vi "main.vi"() -> ()   [LabVIEW 2021]
uses:
  Sources/Plotting-Axis.ctl
  VNA_DataType.ctl
  GEN_States.ctl
  Sources/Data_Cluster.ctl
  Sources/Measurement_Cluster.ctl
  Sources/Mode_Enum.ctl
  Library/TerminalDef.ctl
  <vilib>/Utility/config.llb/Config Data RefNum.ctl
  e59eb776-c2e1-4916-866f-0ee3ec66ac1c.vi
  <vilib>/Utility/config.llb/NI_LVConfig.lvlib
  Library/LibDan.lvlib
panel:
  in  "Control Tab":enum32{"General"}(tab)
  in  "S22Param":enum16{"S11", "S21", "S12", "S22"}(ring)=enum."S22"
  in  "S12Param":enum16{"S11", "S21", "S12", "S22"}(ring)=enum."S12"
  in  "S21Param":enum16{"S11", "S21", "S12", "S22"}(ring)=enum."S21"
  in  "Ramp Dir.":bool=TRUE
  in  "End B (T)":dbl
  in  "Delta B (T)":dbl
  in  "1/s":dbl
  in  "Measure Mode":enum32{"Deltat", "DeltaT", "dB"}(radio)
  in  "Stop @ T/B":bool=TRUE
  out "Temperature (K)":dbl
  out "Mag. Field (T)":dbl
  in  "Log Prefix":string="VNALog"
  in  "Data Type S22":T1
  in  "Data Type S12":T1
  in  "Data Type S21":T1
  in  "Data Type S11":T1
  in  "S22Bool":bool
  in  "S12Bool":bool
  in  "S21Bool":bool
  in  "S11Bool":bool
  in  "End T (K)":dbl
  in  "Delta T (K)":dbl
  in  "StopM_Button":bool
  in  "Log_Button":bool
  in  "Measure_Button":bool
  out "Global B":bool
  out "Global T":bool
  out "Logging":bool
  out "Measuring":bool
  in  "Global T VarRef":refnum<k21>
  in  "Global B VarRef":refnum<k21>
  in  "S11Param":enum16{"S11", "S21", "S12", "S22"}(ring)
  in  "Display Tab":T2(tab)
  out "Terminal":string
  in  "Clear_Button":bool
  in  "Y-Axis":T3=enum."Temperature"
  in  "X-Axis":T3
  out "Test Graph":cluster{"X":dbl, "Y":dbl}[](graph)
  in  "Max Elements":i32=5000
  out "Parameter Plots":cluster{"Ramp Pattern":dbl[], "VNA S22":dbl[]}(graph)
  in  "Param":enum16{"S11", "S21", "S12", "S22"}(ring)
  in  "Following":enum32{"Mag", "Temp", "Last"}(radio)=enum."Last"
  in  "Exit_Button":bool
  # "Parameter"
  # "Data Type"
  # "On/Off"
  # "S12"
  # "S22"
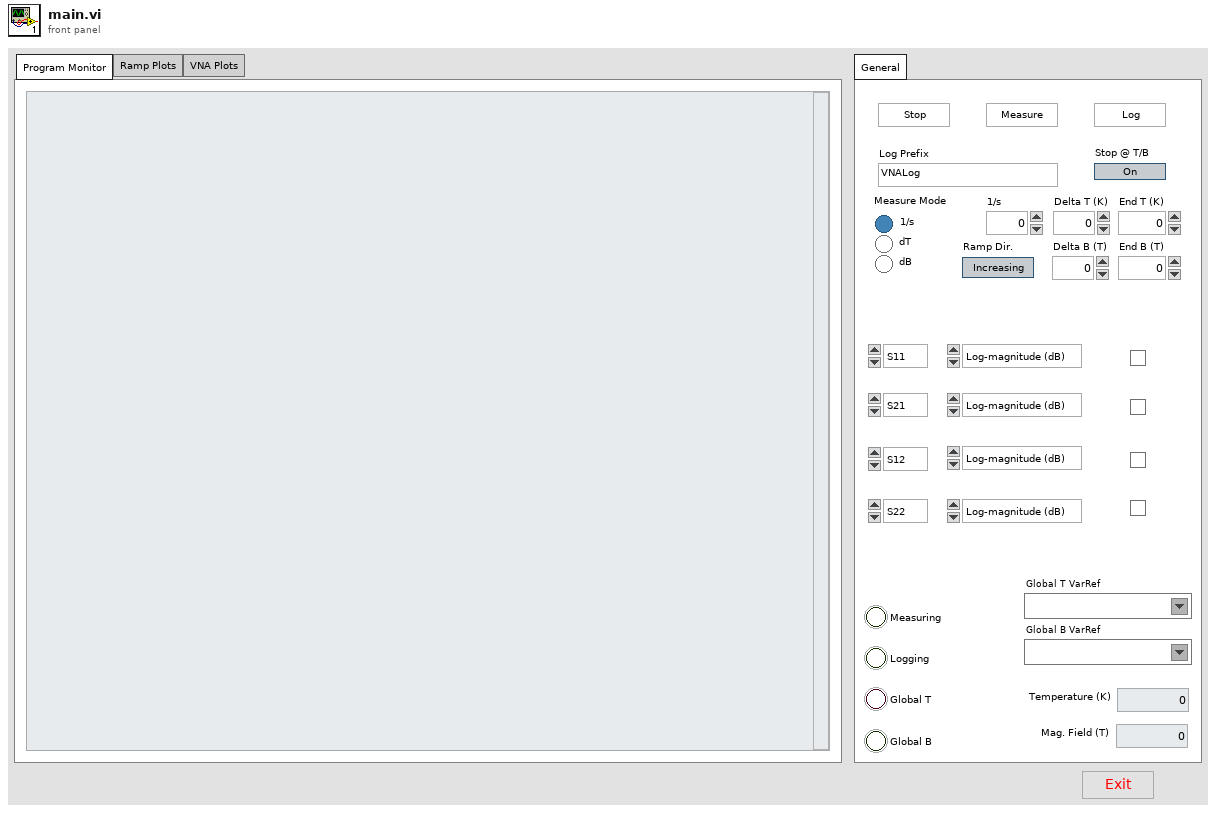
[diagram p1: front panel]
types:
  T1 = typedef "VNA_DataType.ctl" = enum16{"Log-magnitude (dB)", "Linear magnitude", "Phase (deg)", "Time Domain", "Real", "Imaginary", "Group Delay", "Polarlinear"}
  T2 = enum32{"Program Monitor", "Ramp Plots", "VNA Plots"}
  T3 = typedef "Plotting-Axis.ctl" = enum16{"Time", "Temperature", "Magnetic Field"}
  T4 = cluster{"Name":string, "Map":map{string, string}}
  T5 = typedef "LibDan.lvlib/TerminalDef.ctl" = cluster{"Terminal":cluster{"Data":string, "Prompt":string, "Output Refnum":refnum<vi>, "Input":string, "Input Refnum":refnum<vi>}, "TCP":cluster{"HostIP":string, "ServiceName":string, "Port":u16, "Timeout":i32, "TCP ID":refnum<k5>, "TCPConID":refnum<k5>, "Listening?":bool, "ClientCon?":bool}, "Config":cluster{"Path":path, "PathRef":T6, "NewFile?":bool, "Sections":cluster{"Name":string, "Map":map{string, string}}[]}}
  T6 = typedef "NI_LVConfig.lvlib/Config Data RefNum.ctl" = refnum<k1>
  T7 = typedef "Data_Cluster.ctl" = cluster{"Value":dbl, "GUI Data Cluster":cluster{"S11":bool, "S21":bool, "S12":bool, "S22":bool, "S11Meas":enum16{"Log-magnitude (dB)", "Linear magnitude", "Phase (deg)", "Time Domain", "Real", "Imaginary", "Group Delay", "Polarlinear"}, "S21Meas":enum16{"Log-magnitude (dB)", "Linear magnitude", "Phase (deg)", "Time Domain", "Real", "Imaginary", "Group Delay", "Polarlinear"}, "S12Meas":enum16{"Log-magnitude (dB)", "Linear magnitude", "Phase (deg)", "Time Domain", "Real", "Imaginary", "Group Delay", "Polarlinear"}, "S22Meas":enum16{"Log-magnitude (dB)", "Linear magnitude", "Phase (deg)", "Time Domain", "Real", "Imaginary", "Group Delay", "Polarlinear"}, "S11Param":enum16{"S11", "S21", "S12", "S22"}, "S21Param":enum16{"S11", "S21", "S12", "S22"}, "S12Param":enum16{"S11", "S21", "S12", "S22"}, "S22Param":enum16{"S11", "S21", "S12", "S22"}}, "Timing":cluster{"Last Operation":dbl, "Stop @ T/B":bool, "Last Temp":dbl, "Last Mag":dbl, "Ramp Param":cluster{"End T (K)":dbl, "Delta T (K)":dbl, "End B (T)":dbl, "Delta B (T)":dbl}, "LastOp?":bool, "FirstOp?":bool}, "Measurements":T8[], "Hardware":cluster{"VNA TCP Con":refnum<k5>, "VNA TCP Port":i32, "Global T VAR":refnum<k21>, "Global B VAR":refnum<k21>}, "Operation":cluster{"Operation Mode":T9, "Log Folder":path, "Measure Mode":enum32{"Deltat", "DeltaT", "dB"}}}
  T8 = typedef "Measurement_Cluster.ctl" = cluster{"Time Stamp":timestamp, "Temp T":dbl, "Mag B":dbl, "VNA S11":dbl[], "VNA S21":dbl[], "VNA S12":dbl[], "VNA S22":dbl[], "SweepParamArray":cluster{"Start f":dbl, "Stop f":dbl, "Pnts":i32, "Step f":dbl}[]}
  T9 = typedef "Mode_Enum.ctl" = enum16{"Logging", "Idle-Off", "Idle"}
  T10 = typedef "GEN_States.ctl" = enum16{"ClearBuffers", "SwitchToMeas", "SwitchToLog", "SwitchToOff", "Disconnect", "ExitSafe", "RefreshPlotMUnits", "UpdatePlots", "RefreshMUnits", "Read/WriteAll", "InitGUI", "Idle", "ProgInit", "Connect", "ConnectFail"}
  T11 = cluster{"Name":string, "Map":map{string, string}}[]
  T12 = enum16{"Standard", "Buffered", "CRLF", "Immediate"}
  T13 = cluster{"End T (K)":dbl, "Delta T (K)":dbl, "End B (T)":dbl, "Delta B (T)":dbl}
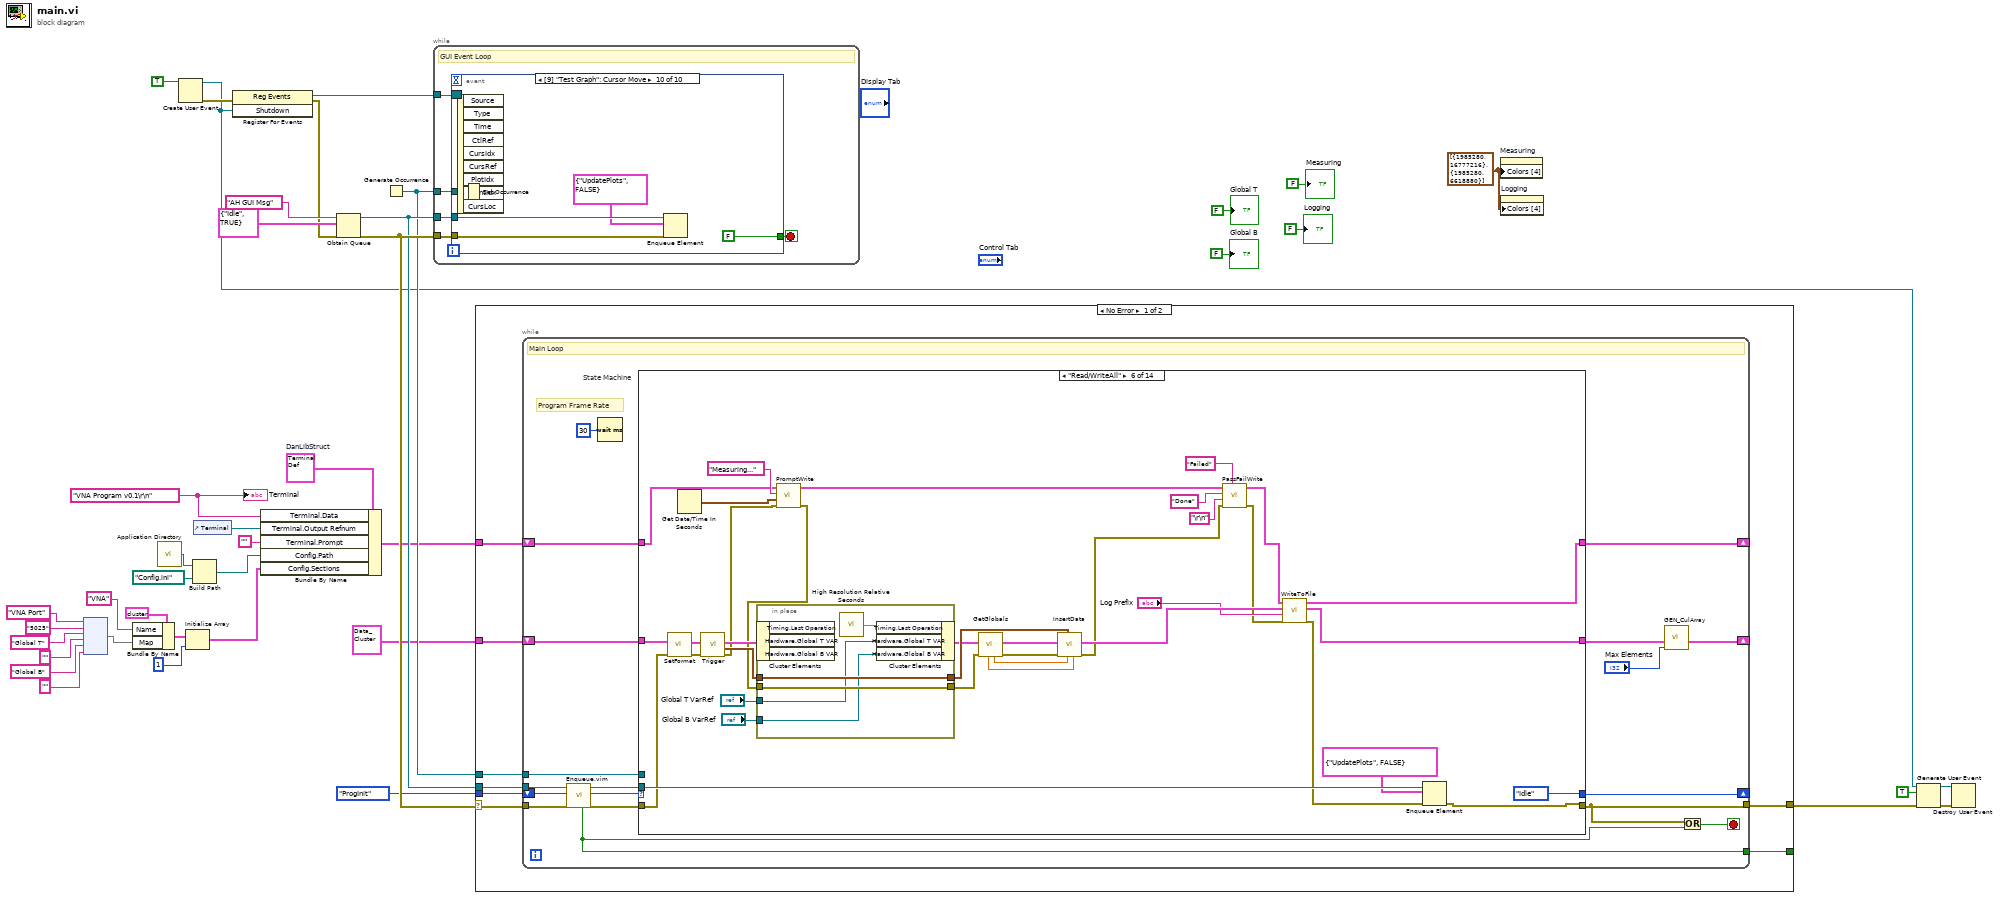
[diagram p0: block diagram]
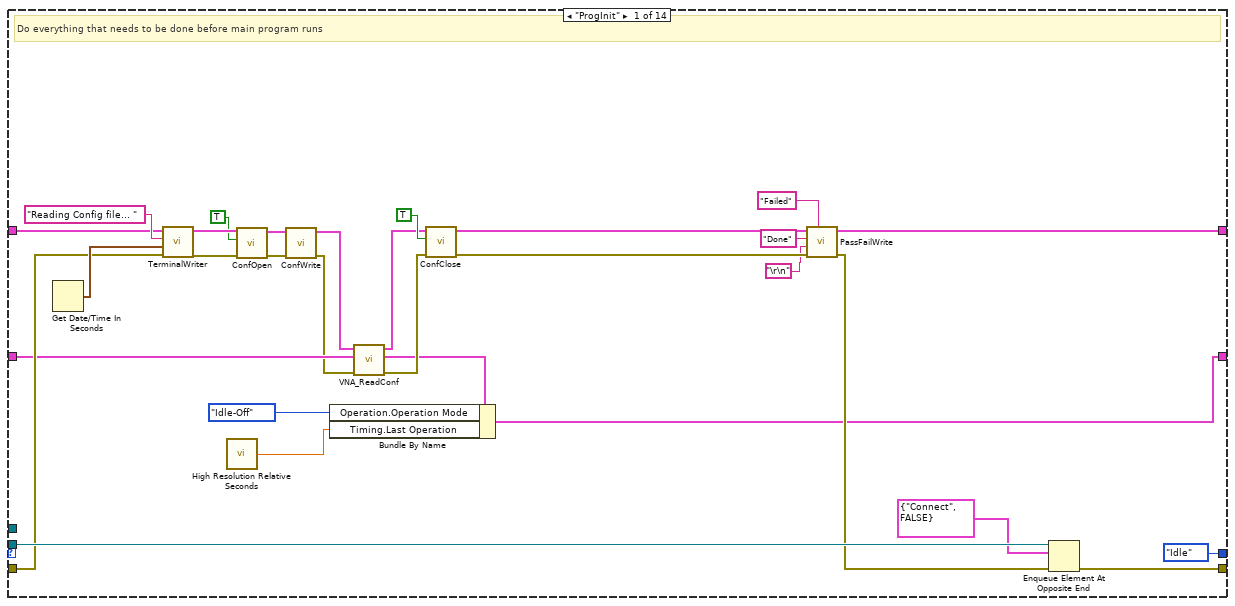
[diagram p2: hidden frame]
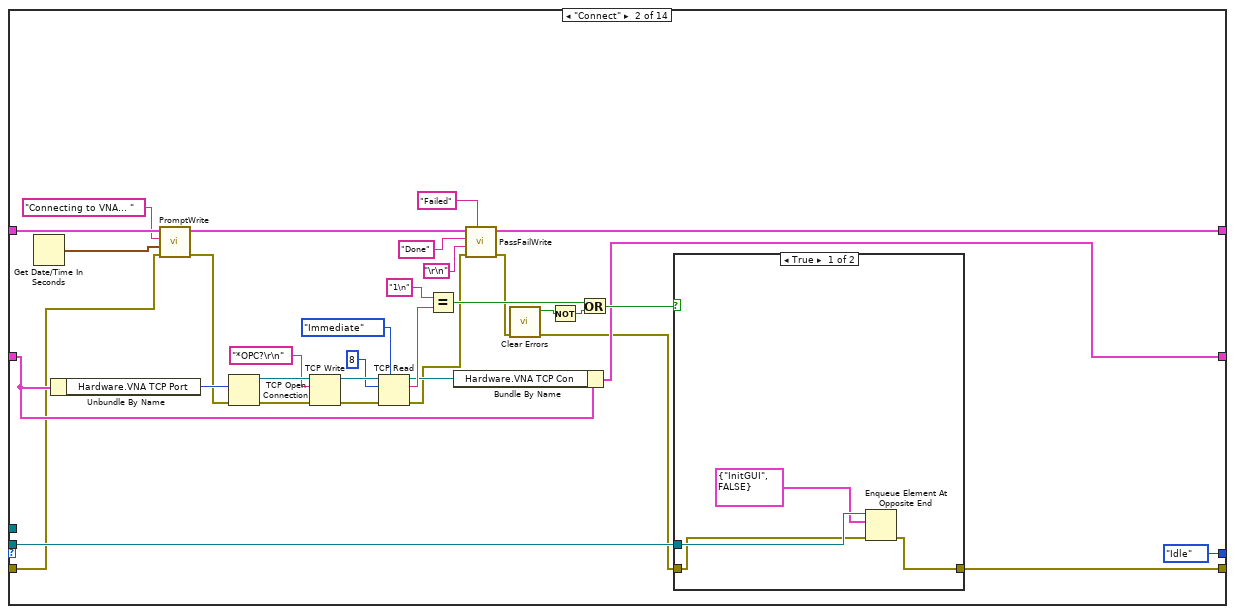
[diagram p3: hidden frame]
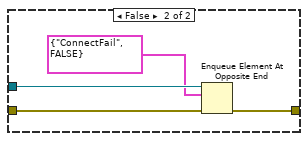
[diagram p4: hidden frame]
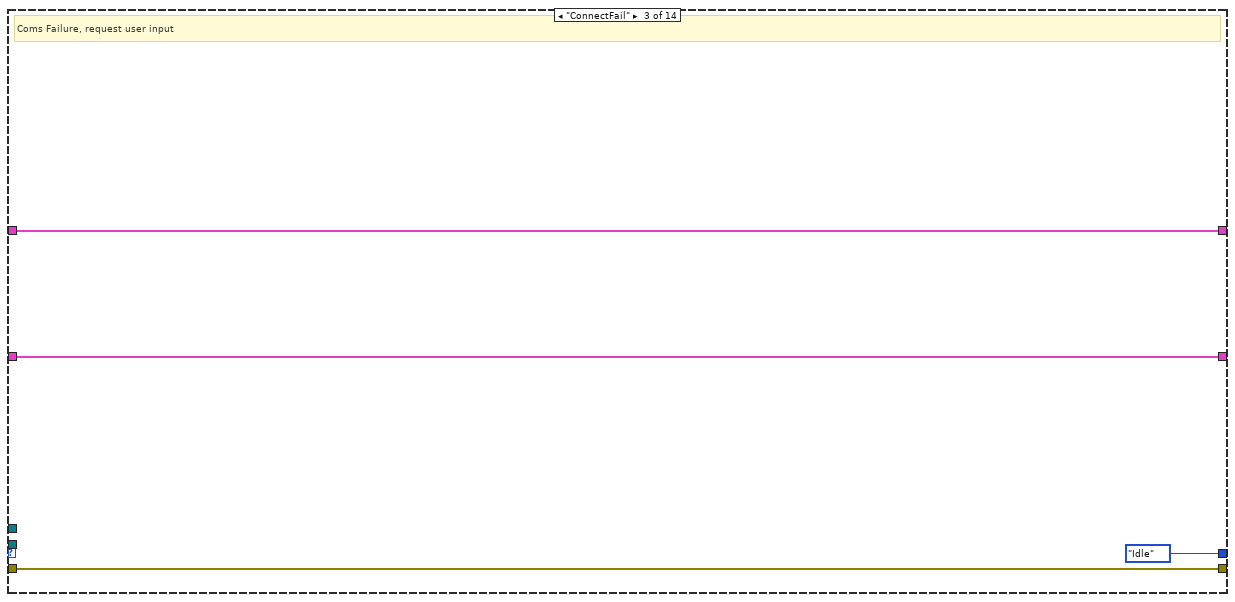
[diagram p5: hidden frame]
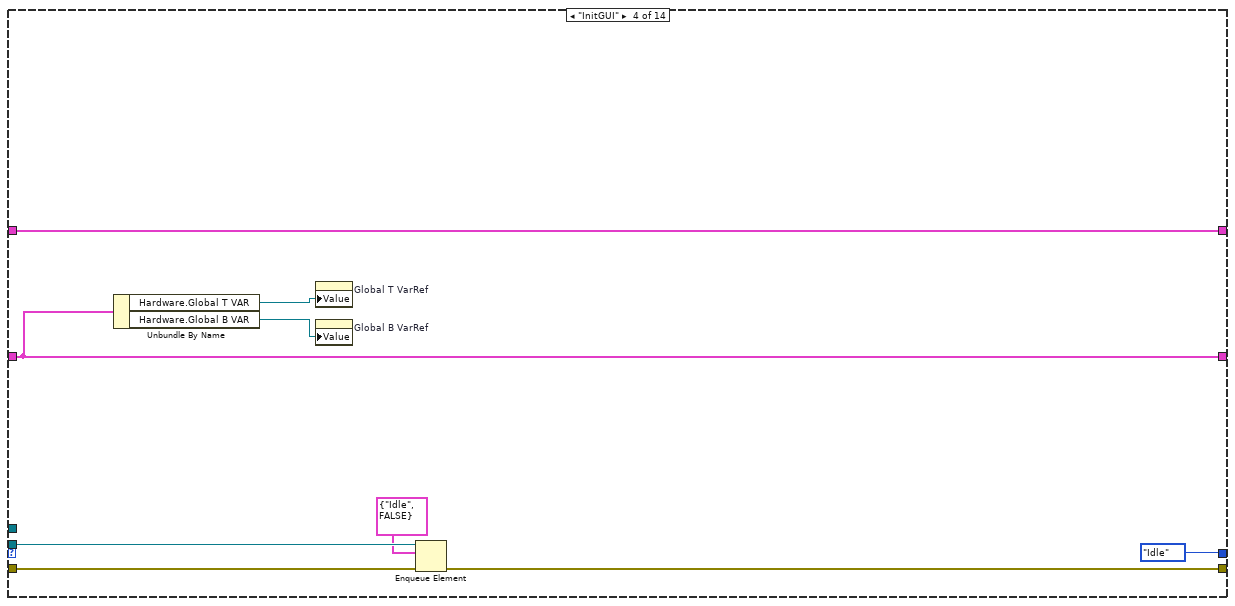
[diagram p6: hidden frame]
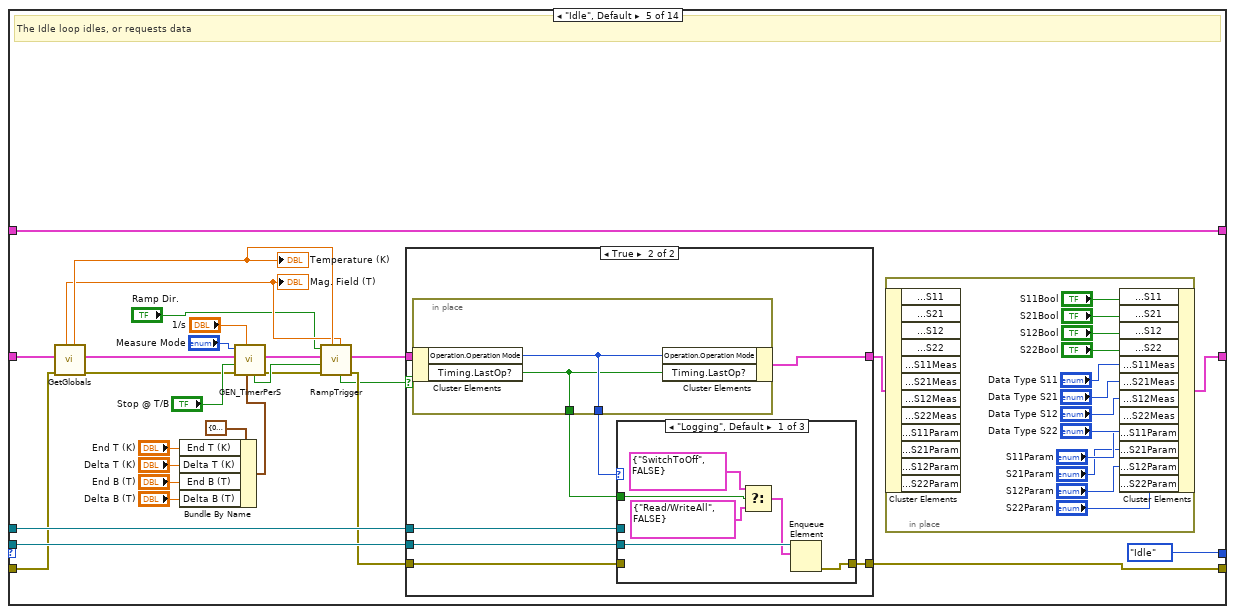
[diagram p7: hidden frame]
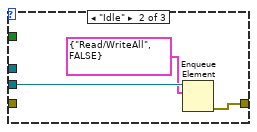
[diagram p9: hidden frame]
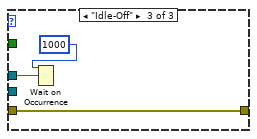
[diagram p10: hidden frame]
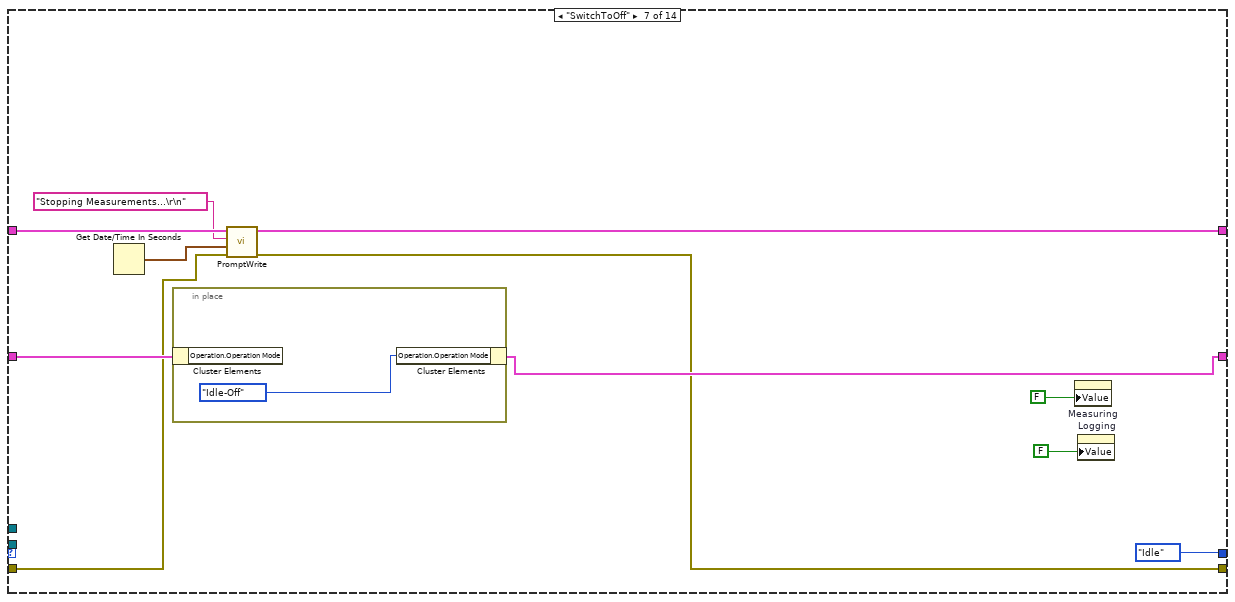
[diagram p11: hidden frame]
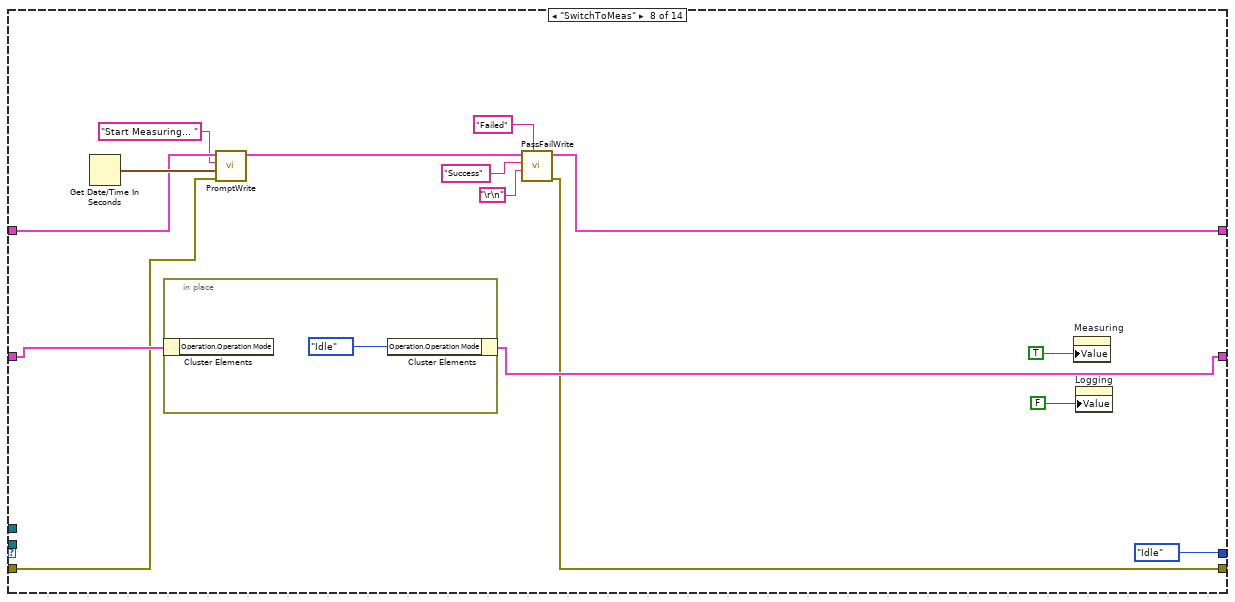
[diagram p12: hidden frame]
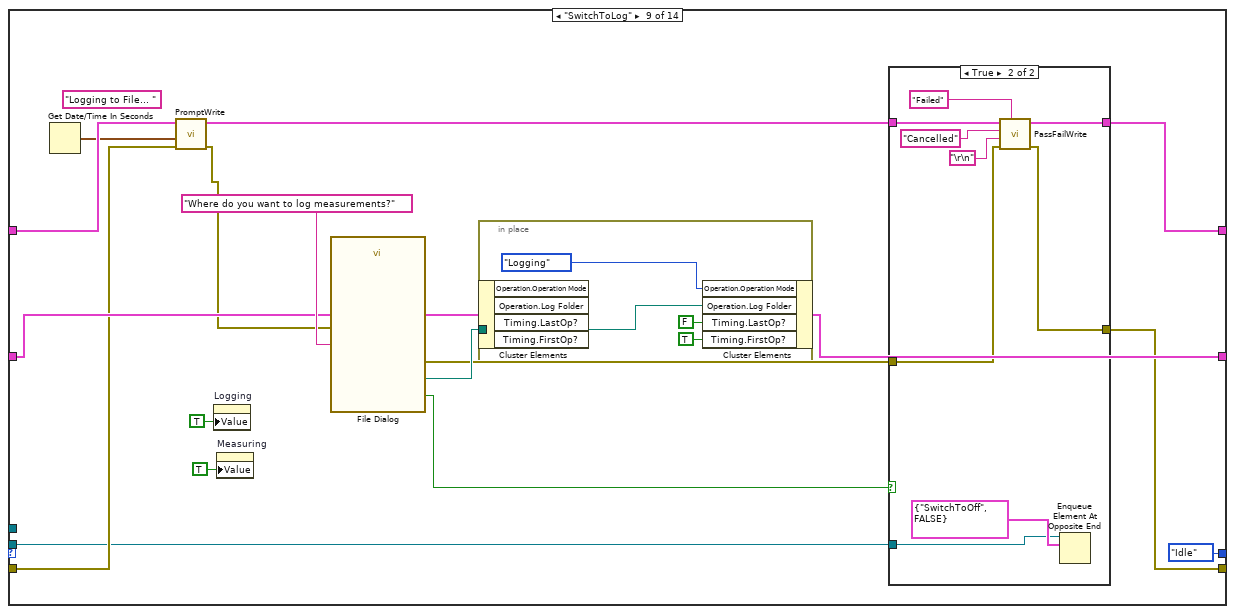
[diagram p13: hidden frame]
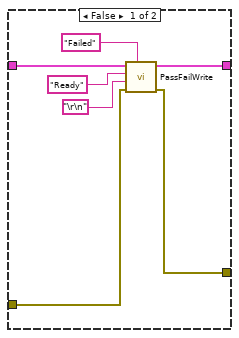
[diagram p14: hidden frame]
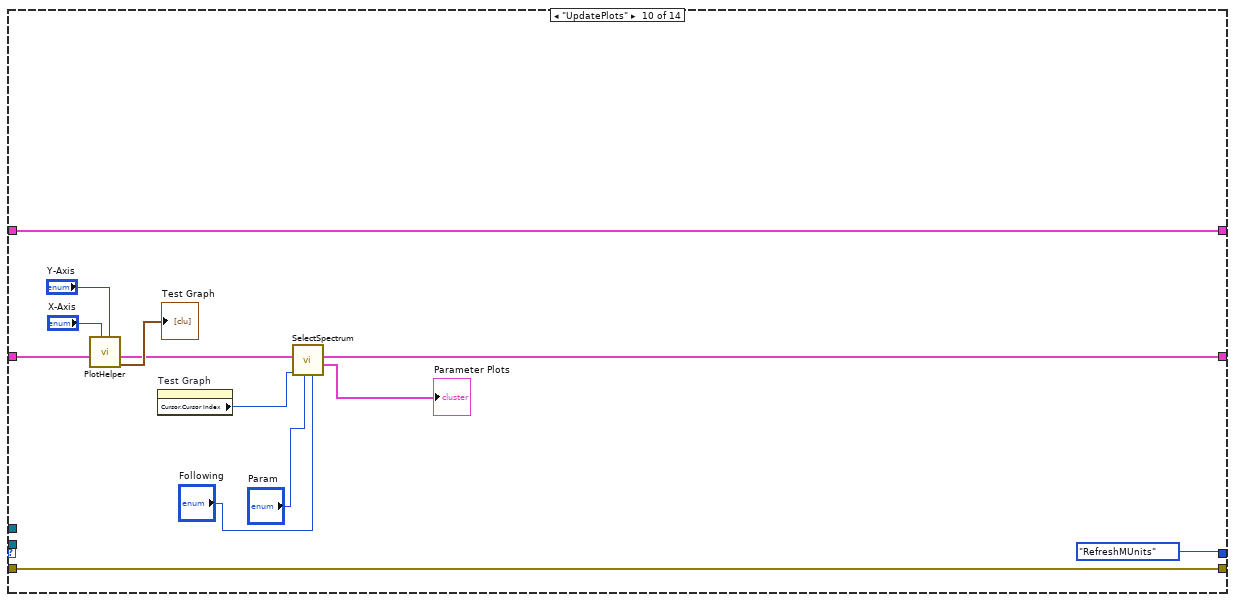
[diagram p15: hidden frame]
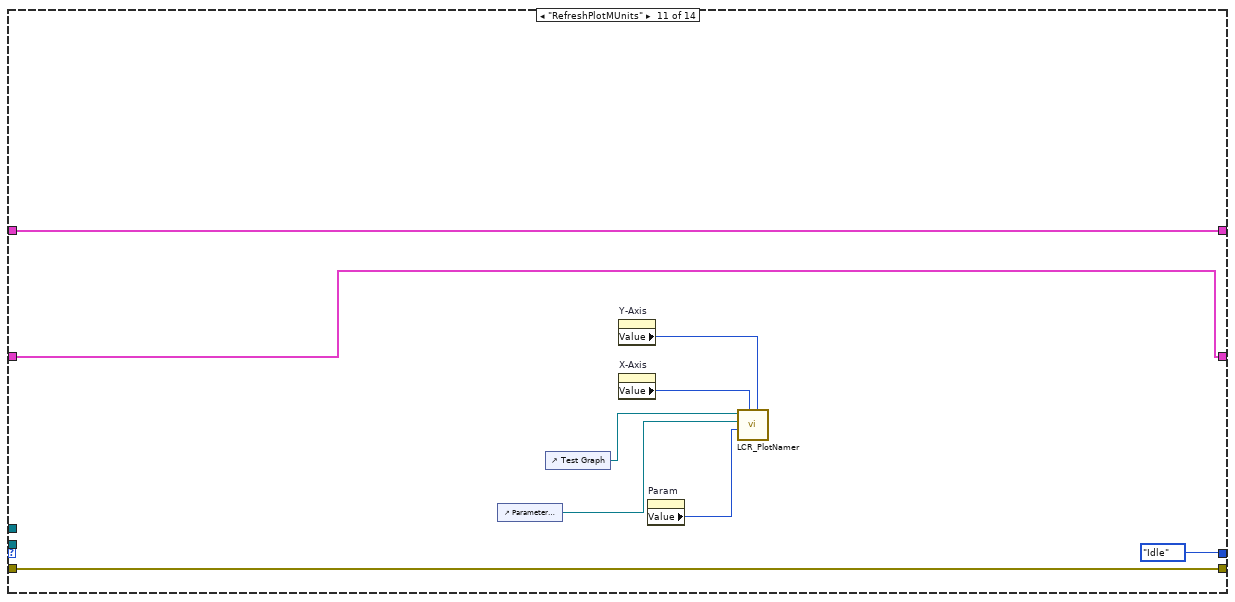
[diagram p16: hidden frame]
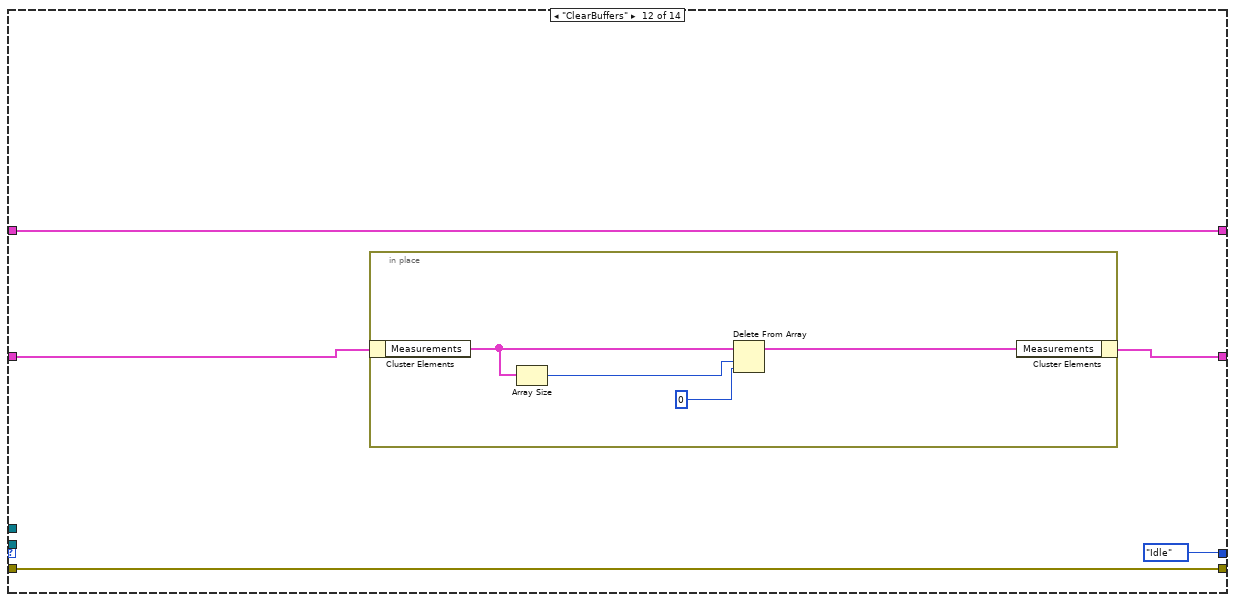
[diagram p17: hidden frame]
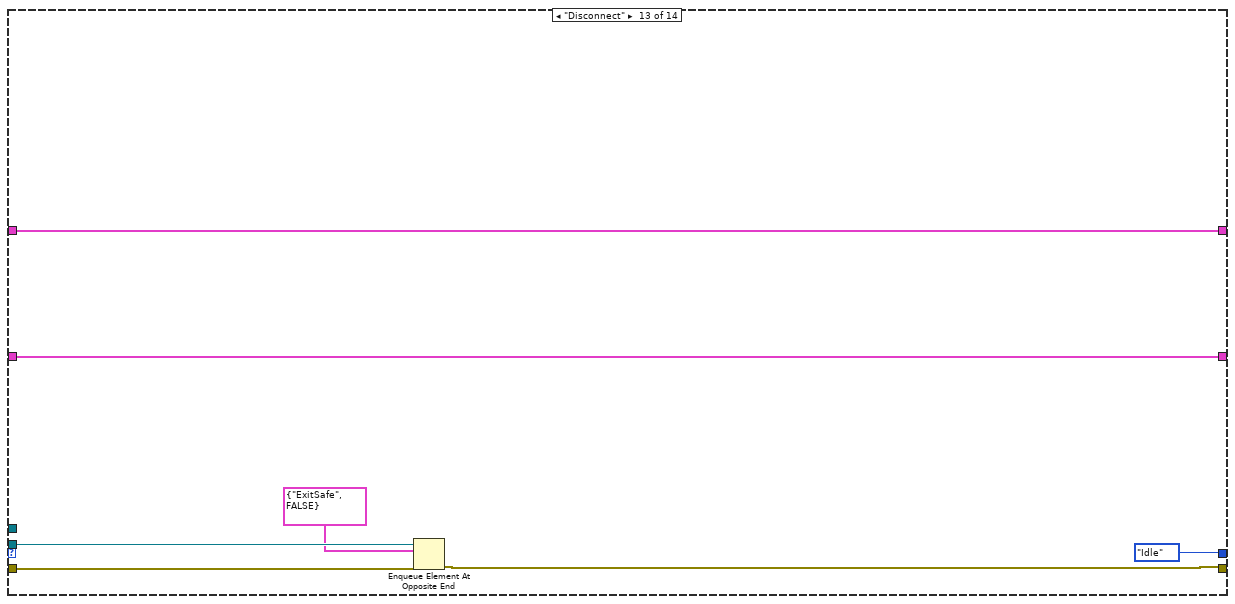
[diagram p18: hidden frame]
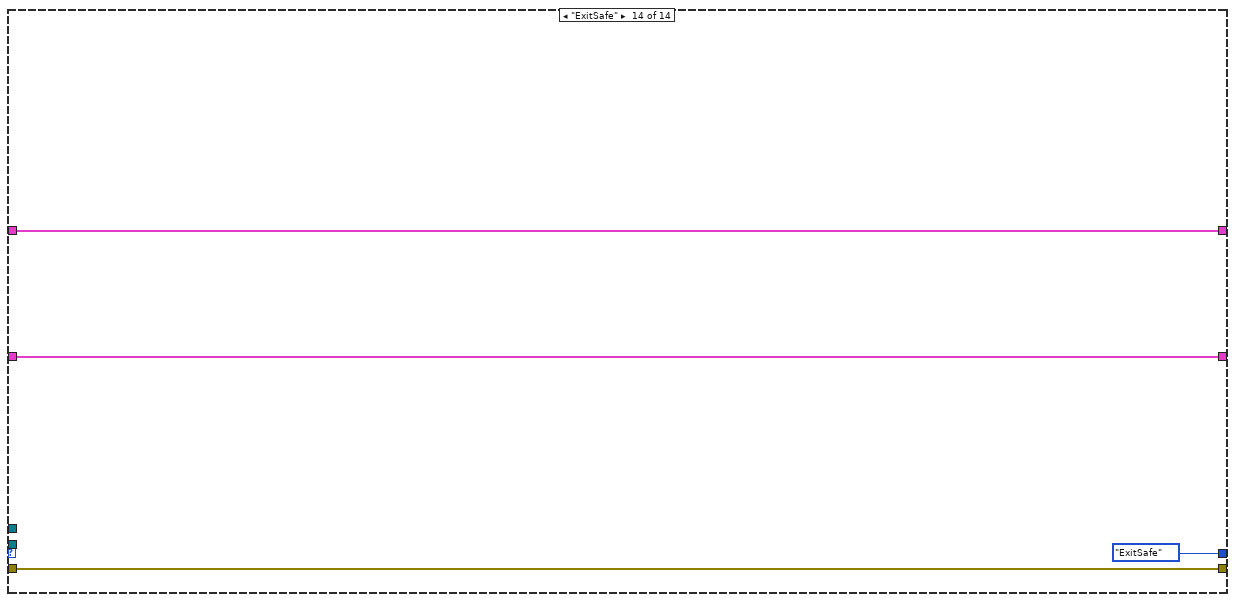
[diagram p19: hidden frame]
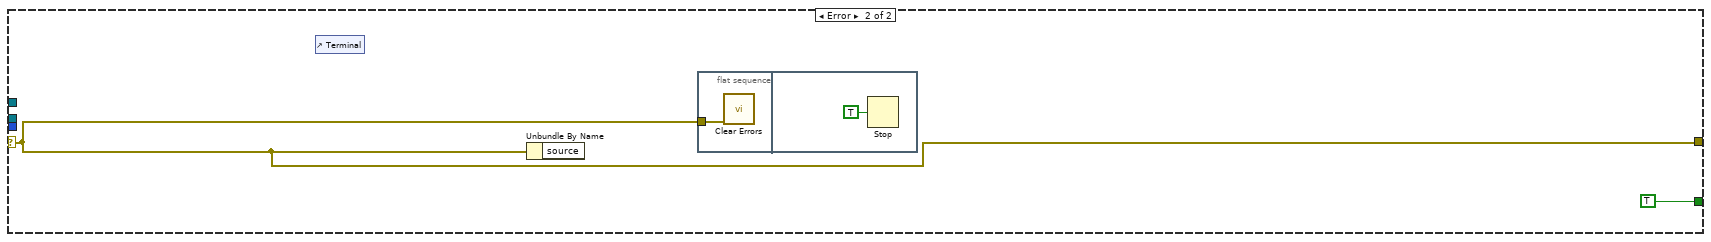
[diagram p20: hidden frame]
diagram:
  w19 = "VNA Program v0.1\r\n"
  w20 = T5 {"Terminal"={"Data"="", "Prompt"="", "Output Refnum"=refnum, "Input"="", "Input Refnum"=refnum}, "TCP"={"HostIP"="", "ServiceName"="", "Port"=0, "Timeout"=0, "TCP ID"=refnum, "TCPConID"=refnum, "Listening?"=FALSE, "ClientCon?"=FALSE}, "Config"={"Path"=path "", "PathRef"=refnum, "NewFile?"=FALSE, "Sections"=[]}}  # DanLibStruct
  w31 = cluster{u32, u32}[] [{1985280, 16777216}, {1985280, 6618880}] ("Colors [4]")
  n1 = node("VNA Port" ("key"), "5025", "Global T" ("key"), "", "Global B", "") -> (w1:map{string, string})
  n2 = Bundle By Name(cluster=T4 {"Name"="", "Map"={}} ("Cluster"), "Name"="VNA", "Map"=w1) -> (w13:T4)
  n3 = call <vilib>:"Application Directory.vi"() -> ("Application Directory"=w16:path)
  n4 = Create User Event(user event datatype=TRUE ("Shutdown")) -> (user event=w21:refnum<user-event>, error out=w28:errorcluster)  [unwired: 1 in]
  n5 = Initialize Array(w13, 1 ("dimension size")) -> (w10:T11)
  n6 = Build Path(base path=w16, name or relative path=path "Config.ini") -> (appended path=w14:path)
  n7 = control-ref of="Terminal"() -> (w18:refnum<vi>)
  n8 = register-events(error in=w28, w21) -> (reference out=w27:refnum<event-registration>, error out=w26:errorcluster)  [unwired: 1 in]
  n9 = Bundle By Name(cluster=w20, "Terminal.Data"=w19, "Terminal.Output Refnum"=w18, "Terminal.Prompt"="", "Config.Path"=w14, "Config.Sections"=w10) -> (w8:T5)
  n10 = Obtain Queue(name (unnamed)="AH GUI Msg", element data type=cluster{T10, bool} {enum."Idle", TRUE}, error in (no error)=w26) -> (queue out=w38:refnum<queue>, error out=w39:errorcluster)  [unwired: 2 in, 1 out]
  n11 = Generate Occurrence() -> (w36:refnum<k4>)
  n12 = while {
    tunnel: w38 -> [w46]
    tunnel: w39 -> [w45]
    tunnel: w36 -> [w43]
    tunnel: w27 -> [w42]
    stop <- w44 stop-if-true
    # "GUI Event Loop"
    n13 = event shown="[9] \"Test Graph\": Cursor Move" {
      selector: w42 -> [_ _ _ _ _ _ _ _ _ _]
      dyn-events: _ -> [_ _ _ _ _ _ _ _ _ _]
      timeout: _ -> [_ _ _ _ _ _ _ _ _ _]
      tunnel: w46 -> [_ w51 w56 w61 w66 w71 w76 w81 w86 w91]
      tunnel: w45 -> [_ w50 w55 w60 w65 w70 w75 w80 w85 w90]
      tunnel: [_ TRUE FALSE FALSE FALSE FALSE FALSE FALSE FALSE FALSE] -> w44
      tunnel: w43 -> [_ w47 w52 w57 w62 w67 w73 w78 w83 w88]
      event Timeout {
        n14 = event-data() -> ()  [unwired: 1 in, 3 out]
      }
      event "Exit_Button": Value Change {
        n15 = event-data() -> ()  [unwired: 1 in, 6 out]
        n16 = Set Occurrence(w47) -> ()
        n17 = Enqueue Element At Opposite End(queue=w51, element=cluster{T10, bool} {enum."ExitSafe", TRUE}, error in (no error)=w50) -> ()  [unwired: 1 in, 3 out]
      }
      event "StopM_Button": Value Change {
        n18 = event-data() -> ()  [unwired: 1 in, 6 out]
        n19 = Set Occurrence(w52) -> ()
        n20 = Enqueue Element(queue=w56, element=cluster{T10, bool} {enum."SwitchToOff", FALSE}, error in (no error)=w55) -> ()  [unwired: 1 in, 3 out]
      }
      event "Measure_Button": Value Change {
        n21 = event-data() -> ()  [unwired: 1 in, 6 out]
        n22 = Set Occurrence(w57) -> ()
        n23 = Enqueue Element(queue=w61, element=cluster{T10, bool} {enum."SwitchToMeas", FALSE}, error in (no error)=w60) -> ()  [unwired: 1 in, 3 out]
      }
      event "Log_Button": Value Change {
        n24 = event-data() -> ()  [unwired: 1 in, 6 out]
        n25 = Set Occurrence(w62) -> ()
        n26 = Enqueue Element(queue=w66, element=cluster{T10, bool} {enum."SwitchToLog", FALSE}, error in (no error)=w65) -> ()  [unwired: 1 in, 3 out]
      }
      event "Clear_Button": Value Change {
        n27 = event-data() -> ()  [unwired: 1 in, 6 out]
        n28 = Set Occurrence(w67) -> ()
        n29 = Enqueue Element(queue=w71, element=cluster{T10, bool} {enum."ClearBuffers", FALSE}, error in (no error)=w70) -> ()  [unwired: 1 in, 3 out]
      }
      event Value Change {
        n30 = event-data() -> ()  [unwired: 1 in, 6 out]
        n31 = Set Occurrence(w73) -> ()
        n32 = Enqueue Element(queue=w76, element=cluster{T10, bool} {enum."RefreshPlotMUnits", FALSE}, error in (no error)=w75) -> ()  [unwired: 1 in, 3 out]
      }
      event "Param": Value Change {
        n33 = event-data() -> ()  [unwired: 1 in, 6 out]
        n34 = Set Occurrence(w78) -> ()
        n35 = Enqueue Element(queue=w81, element=cluster{T10, bool} {enum."UpdatePlots", FALSE}, error in (no error)=w80) -> ()  [unwired: 1 in, 3 out]
      }
      event "Following": Value Change {
        n36 = event-data() -> ()  [unwired: 1 in, 6 out]
        n37 = Set Occurrence(w83) -> ()
        n38 = Enqueue Element(queue=w86, element=cluster{T10, bool} {enum."UpdatePlots", FALSE}, error in (no error)=w85) -> ()  [unwired: 1 in, 3 out]
      }
      event "Test Graph": Cursor Move {
        n39 = event-data() -> ()  [unwired: 1 in, 9 out]
        n40 = Set Occurrence(w88) -> ()
        n41 = Enqueue Element(queue=w91, element=cluster{T10, bool} {enum."UpdatePlots", FALSE}, error in (no error)=w90) -> ()  [unwired: 1 in, 3 out]
      }
    }
  }
  n42 = case shown="No Error" w39 {
    selector: w39 -> [w99 w415]
    tunnel: w38 -> [w98 _]
    tunnel: GEN_States."ProgInit" ("State") -> [w97 _]
    tunnel: [w93 TRUE] -> _
    tunnel: T7 {"Value"=0.0, "GUI Data Cluster"={"S11"=FALSE, "S21"=FALSE, "S12"=FALSE, "S22"=FALSE, "S11Meas"=enum."Log-magnitude (dB)", "S21Meas"=enum."Log-magnitude (dB)", "S12Meas"=enum."Log-magnitude (dB)", "S22Meas"=enum."Log-magnitude (dB)", "S11Param"=enum."S11", "S21Param"=enum."S21", "S12Param"=enum."S12", "S22Param"=enum."S22"}, "Timing"={"Last Operation"=0.0, "Stop @ T/B"=FALSE, "Last Temp"=0.0, "Last Mag"=0.0, "Ramp Param"={"End T (K)"=0.0, "Delta T (K)"=0.0, "End B (T)"=0.0, "Delta B (T)"=0.0}, "LastOp?"=FALSE, "FirstOp?"=FALSE}, "Measurements"=[], "Hardware"={"VNA TCP Con"=refnum, "VNA TCP Port"=5025, "Global T VAR"="", "Global B VAR"=""}, "Operation"={"Operation Mode"=enum."Logging", "Log Folder"=path "", "Measure Mode"=enum."Deltat"}} -> [w96 _]
    tunnel: w36 -> [w95 _]
    tunnel: [w94 w415] -> w23
    tunnel: w8 -> [w92 _]
    frame No Error {
      n43 = while {
        tunnel: w99 -> [w106]
        tunnel: w98 -> [w108]
        shift-right: [w100] -> _
        shift-left: w97 -> [w102]
        tunnel: [w105] -> w93
        shift-right: [w112] -> _
        shift-left: w96 -> [w115]
        tunnel: w95 -> [w114]
        tunnel: [w110] -> w94
        shift-right: [w103] -> _
        shift-left: w92 -> [w109]
        stop <- w116 stop-if-true
        # "Program Frame Rate"
        # "Main Loop"
        n44 = call "Enqueue.vim"("error in (no error)"=w106, "Variant"=w102, "queue In"=w108) -> ("error out"=w104:errorcluster, "Variant Out"=w101:T10, "queue out"=w107:refnum<queue>, "Exit?"=w105:bool)  [unwired: 5 in]
        n45 = Wait (ms)(milliseconds to wait=u32 30) -> ()  [unwired: 1 out]
        n46 = case "State Machine" shown="\"Read/WriteAll\"" w101 {
          tunnel: w107 -> [w147 w167 _ w201 w229 w302 _ _ w342 _ _ _ w409 _]
          tunnel: w115 -> [w134 w170 w192 w195 w221 w299 w315 w331 w349 w383 w394 w399 w410 w414]
          tunnel: [w118 w163 w192 w195 w223 w282 w314 w330 w348 w374 w394 w398 w410 w414] -> w113
          tunnel: [w127 w161 w190 w196 w228 w293 w308 w320 w337 w379 w388 w396 w404 w411] -> w110
          tunnel: w114 -> [_ _ _ _ w230 _ _ _ _ _ _ _ _ _]
          tunnel: w109 -> [w138 w160 w189 w198 w226 w286 w313 w328 w347 w381 w390 w395 w405 w412]
          tunnel: w104 -> [w137 w157 w190 w197 w222 w297 w310 w326 w345 w379 w388 w396 w406 w411]
          tunnel: [w124 w155 w189 w198 w226 w281 w309 w321 w336 w381 w390 w395 w405 w412] -> w103
          tunnel: [GEN_States."Idle" ("State") GEN_States."Idle" ("State") GEN_States."Idle" ("State") GEN_States."Idle" ("State") GEN_States."Idle" ("State") GEN_States."Idle" ("State") GEN_States."Idle" ("State") GEN_States."Idle" ("State") GEN_States."Idle" ("State") GEN_States."RefreshMUnits" ("State") GEN_States."Idle" ("State") GEN_States."Idle" ("State") GEN_States."Idle" ("State") GEN_States."ExitSafe" ("State")] -> w100
          frame "ProgInit" {
            # "Do everything that needs to be done before main program runs"
            n47 = Get Date/Time In Seconds() -> (seconds since 1Jan1904=w145:timestamp)
            n48 = call-poly "TerminalWriter.vi"("error in"=w137, "time"=w145, "string"="Reading Config file... ", "TerminalIn"=w138) -> ("error out"=w142:errorcluster, "TerminalOut"=w143:T5)  [unwired: 6 in]
            n49 = call <vilib>:"High Resolution Relative Seconds.vi"() -> ("relative seconds"=w128:dbl)
            n50 = call "ConfOpen.vi"("error in"=w142, "create file if necessary (T)"=TRUE, "StructIn"=w143) -> ("error out"=w139:errorcluster, "StructOut"=w140:T5)  [unwired: 6 in, 1 out]
            n51 = call "ConfWrite.vi"("error in"=w139, "StructIn"=w140) -> ("error out"=w133:errorcluster, "StructOut"=w135:T5)  [unwired: 8 in]
            n52 = call "VNA_ReadConf.vi"("error in"=w133, "VNAClusterIn"=w134, "GeneralClusterIn"=w135) -> ("error out"=w132:errorcluster, "VNAClusterOut"=w129:T7, "GeneralClusterOut"=w131:T5)  [unwired: 6 in]
            n53 = Bundle By Name(cluster=w129, "Operation.Operation Mode"=Mode_Enum."Idle-Off", "Timing.Last Operation"=w128) -> (w118:T7)
            n54 = call "ConfClose.vi"("error in"=w132, "Write?"=TRUE, "StructIn"=w131) -> ("error out"=w123:errorcluster, "StructOut"=w125:T5)  [unwired: 7 in]
            n55 = call "PassFailWrite.vi"("FailString"="Failed", "error in"=w123, "End"="\r\n", "PassString"="Done", "TerminalIn"=w125) -> ("error out"=w122:errorcluster, "TerminalOut"=w124:T5)  [unwired: 5 in]
            n56 = Enqueue Element At Opposite End(queue=w147, element=cluster{T10, bool} {enum."Connect", FALSE}, error in (no error)=w122) -> (error out=w127:errorcluster)  [unwired: 1 in, 2 out]
          }
          frame "Connect" {
            n57 = Get Date/Time In Seconds() -> (seconds since 1Jan1904=w158:timestamp)
            n58 = Unbundle By Name(w170) -> ("Hardware.VNA TCP Port"=w180:i32)
            n59 = call "PromptWrite.vi"("error in"=w157, "time"=w158, "string"="Connecting to VNA... ", "TerminalIn"=w160) -> ("error out"=w156:errorcluster, "TerminalOut"=w154:T5)  [unwired: 6 in]
            n60 = TCP Open Connection(remote port or service name=w180, error in (no error)=w156) -> (connection ID=w178:refnum<k5>, error out=w179:errorcluster)  [unwired: 3 in]
            n61 = TCP Write(connection ID=w178, data in="*OPC?\r\n", error in (no error)=w179) -> (connection ID out=w176:refnum<k5>, error out=w175:errorcluster)  [unwired: 1 in, 1 out]
            n62 = TCP Read(connection ID=w176, bytes to read=8, error in (no error)=w175, 7:T12."Immediate" ("mode (standard)")) -> (connection ID out=w169:refnum<k5>, data out=w173:string, error out=w153:errorcluster)  [unwired: 1 in]
            n63 = Equal?(x="1\n", y=w173) -> (x = y?=w171:bool)
            n64 = Bundle By Name(cluster=w170, "Hardware.VNA TCP Con"=w169) -> (w163:T7)
            n65 = call "PassFailWrite.vi"("FailString"="Failed", "error in"=w153, "End"="\r\n", "PassString"="Done", "TerminalIn"=w154) -> ("error out"=w152:errorcluster, "TerminalOut"=w155:T5)  [unwired: 5 in]
            n66 = call <vilib>:"Clear Errors.vi"("error in (no error)"=w152) -> ("error out"=w162:errorcluster, "specific error cleared?"=w166:bool)  [unwired: 5 in]
            n67 = Not(x=w166) -> (.not. x?=w165:bool)
            n68 = Or(x=w171, y=w165) -> (x .or. y?=w164:bool)
            n69 = case shown="True" w164 {
              tunnel: w167 -> [w184 w188]
              tunnel: w162 -> [w182 w186]
              tunnel: [w181 w185] -> w161
              frame True {
                n70 = Enqueue Element At Opposite End(queue=w184, element=cluster{T10, bool} {enum."InitGUI", FALSE}, error in (no error)=w182) -> (error out=w181:errorcluster)  [unwired: 1 in, 2 out]
              }
              frame False {
                n71 = Enqueue Element At Opposite End(queue=w188, element=cluster{T10, bool} {enum."ConnectFail", FALSE}, error in (no error)=w186) -> (error out=w185:errorcluster)  [unwired: 1 in, 2 out]
              }
            }
          }
          frame "ConnectFail" {
            # "Coms Failure, request user input"
          }
          frame "InitGUI" {
            n72 = Unbundle By Name(w195) -> ("Hardware.Global T VAR"=w194:refnum<k21>, "Hardware.Global B VAR"=w193:refnum<k21>)
            n73 = property on="Global T VarRef" class="Variable (strict)"("Value"=w194) -> ()  [unwired: 2 in, 2 out]
            n74 = property on="Global B VarRef" class="Variable (strict)"("Value"=w193) -> ()  [unwired: 2 in, 2 out]
            n75 = Enqueue Element(queue=w201, element=cluster{T10, bool} {enum."Idle", FALSE}, error in (no error)=w197) -> (error out=w196:errorcluster)  [unwired: 1 in, 2 out]
          }
          frame "Idle", Default {
            # "The Idle loop idles, or requests data"
            n76 = call "GetGlobals.vi"("error in (no error)"=w222, "VNACluster In"=w221) -> ("error out"=w219:errorcluster, "VNACluster Out"=w220:T7, "Temp"=w208:dbl, "Mag"=w207:dbl)  [unwired: 6 in]
            "Temperature (K)" <- w208
            "Mag. Field (T)" <- w207
            n77 = Bundle By Name(cluster=T13 {"End T (K)"=0.0, "Delta T (K)"=0.0, "End B (T)"=0.0, "Delta B (T)"=0.0} ("Ramp Param"), "End T (K)"="End T (K)", "Delta T (K)"="Delta T (K)", "End B (T)"="End B (T)", "Delta B (T)"="Delta B (T)") -> (w215:T13)
            n78 = call "GEN_TimerPerS.vi"("Ramp Param"=w215, "1/x"="1/s", "error in"=w219, "Timing.Stop @ T"="Stop @ T/B", "VNACluster In"=w220, "Measure Mode"="Measure Mode") -> ("error out"=w205:errorcluster, "VNACluster Out"=w210:T7, "Time"=w206:bool)  [unwired: 3 in]
            n79 = call "RampTrigger.vi"("Curr B"=w207, "Curr T"=w208, "error in"=w205, "dt Trig"=w206, "VNACluster In"=w210, "Ramp Dir"="Ramp Dir.") -> ("error out"=w204:errorcluster, "VNACluster Out"=w209:T7, "Trigger"=w203:bool)  [unwired: 3 in]
            n80 = case shown="True" w203 {
              tunnel: w230 -> [_ w252]
              tunnel: w229 -> [_ w251]
              tunnel: [w244 w250] -> w228
              tunnel: w204 -> [w244 w249]
              tunnel: w209 -> [w243 w248]
              tunnel: [w243 w247] -> w224
              frame False {
              }
              frame True {
                n81 = in-place {
                  in-place-border: [w254] -> w246
                  in-place-border: [w253] -> w245
                  n82 = in-place-cluster #1(w248) -> ("Operation.Operation Mode"=w254:T9, "Timing.LastOp?"=w253:bool)
                  n83 = in-place-cluster #1("Operation.Operation Mode"=w254, "Timing.LastOp?"=w253) -> (w247:T7)
                }
                n84 = case shown="\"Logging\", Default" w246 {
                  tunnel: w252 -> [_ _ w266]
                  tunnel: w251 -> [w260 w263 _]
                  tunnel: [w259 w261 w264] -> w250
                  tunnel: w249 -> [_ _ w264]
                  tunnel: w245 -> [w258 _ _]
                  frame "Logging", Default {
                    n85 = Select(t=cluster{T10, bool} {enum."SwitchToOff", FALSE} ("element"), s=w258, f=cluster{T10, bool} {enum."Read/WriteAll", FALSE} ("element")) -> (s? t:f=w255:cluster{T10, bool})
                    n86 = Enqueue Element(queue=w260, element=w255) -> (error out=w259:errorcluster)  [unwired: 2 in, 2 out]
                  }
                  frame "Idle" {
                    n87 = Enqueue Element(queue=w263, element=cluster{T10, bool} {enum."Read/WriteAll", FALSE}) -> (error out=w261:errorcluster)  [unwired: 2 in, 2 out]
                  }
                  frame "Idle-Off" {
                    n88 = Wait on Occurrence(2:w266, 3:1000 ("ms timeout (-1)")) -> ()  [unwired: 1 in, 1 out]
                  }
                }
              }
            }
            n89 = in-place {
              n90 = in-place-cluster #2(w224) -> ()  [unwired: 12 out]
              n91 = in-place-cluster #2("GUI Data Cluster.S11"="S11Bool", "GUI Data Cluster.S21"="S21Bool", "GUI Data Cluster.S12"="S12Bool", "GUI Data Cluster.S22"="S22Bool", "GUI Data Cluster.S11Meas"="Data Type S11", "GUI Data Cluster.S21Meas"="Data Type S21", "GUI Data Cluster.S12Meas"="Data Type S12", "GUI Data Cluster.S22Meas"="Data Type S22", "GUI Data Cluster.S11Param"="S11Param", "GUI Data Cluster.S21Param"="S21Param", "GUI Data Cluster.S12Param"="S12Param", "GUI Data Cluster.S22Param"="S22Param") -> (w223:T7)
            }
          }
          frame "Read/WriteAll" {
            n92 = call "SetFormat.vi"("error in (no error)"=w297, "VNACluster In"=w299) -> ("error out"=w269:errorcluster, "VNACluster Out"=w300:T7)  [unwired: 7 in, 1 out]
            n93 = Get Date/Time In Seconds() -> (seconds since 1Jan1904=w291:timestamp)
            n94 = call "Trigger.vi"("error in (no error)"=w269, "VNACluster In"=w300) -> ("error out"=w268:errorcluster, "TriggerTime"=w296:timestamp, "VNACluster Out"=w298:T7)  [unwired: 7 in]
            n95 = call "PromptWrite.vi"("error in"=w268, "time"=w291, "string"="Measuring...", "TerminalIn"=w286) -> ("error out"=w267:errorcluster, "TerminalOut"=w290:T5)  [unwired: 6 in]
            n96 = in-place {
              in-place-border: w296 -> [w306]
              in-place-border: w267 -> [w305]
              in-place-border: [w306] -> w295
              in-place-border: [w305] -> w273
              in-place-border: "Global B VarRef" -> [w304]
              in-place-border: "Global T VarRef" -> [w303]
              n97 = in-place-cluster #3(w298) -> ()  [unwired: 3 out]
              n98 = call <vilib>:"High Resolution Relative Seconds.vi"() -> ("relative seconds"=w307:dbl)
              n99 = in-place-cluster #3("Timing.Last Operation"=w307, "Hardware.Global T VAR"=w303, "Hardware.Global B VAR"=w304) -> (w274:T7)
            }
            n100 = call "GetGlobals.vi"("error in (no error)"=w273, "VNACluster In"=w274) -> ("error out"=w272:errorcluster, "VNACluster Out"=w275:T7, "Temp"=w271:dbl, "Mag"=w270:dbl)  [unwired: 6 in]
            n101 = call "InsertData.vi"("Mag B"=w270, "Temp T"=w271, "Time Stamp"=w295, "error in (no error)"=w272, "VNACluster In"=w275) -> ("error out"=w279:errorcluster, "VNACluster Out"=w283:T7)  [unwired: 5 in]
            n102 = call "PassFailWrite.vi"("FailString"="Failed", "error in"=w279, "End"="\r\n", "PassString"="Done", "TerminalIn"=w290) -> ("error out"=w278:errorcluster, "TerminalOut"=w285:T5)  [unwired: 5 in]
            n103 = call "WriteToFile.vi"("error in"=w278, "Log Prefix"="Log Prefix", "VNACluster In"=w283, "TerminalIn"=w285) -> ("error out"=w284:errorcluster, "VNACluster Out"=w282:T7, "TerminalOut"=w281:T5)  [unwired: 5 in]
            n104 = Enqueue Element(queue=w302, element=cluster{T10, bool} {enum."UpdatePlots", FALSE}, error in (no error)=w284) -> (error out=w293:errorcluster)  [unwired: 1 in, 2 out]
          }
          frame "SwitchToOff" {
            n105 = Get Date/Time In Seconds() -> (seconds since 1Jan1904=w312:timestamp)
            n106 = in-place {
              n107 = in-place-cluster #4(w315) -> ()  [unwired: 1 out]
              n108 = in-place-cluster #4("Operation.Operation Mode"=Mode_Enum."Idle-Off") -> (w314:T7)
            }
            n109 = call "PromptWrite.vi"("error in"=w310, "time"=w312, "string"="Stopping Measurements...\r\n", "TerminalIn"=w313) -> ("error out"=w308:errorcluster, "TerminalOut"=w309:T5)  [unwired: 6 in]
            n110 = property on="Measuring" class="Bool (strict)"("Value"=FALSE ("Measuring")) -> ()  [unwired: 2 in, 2 out]
            n111 = property on="Logging" class="Bool (strict)"("Value"=FALSE ("Logging")) -> ()  [unwired: 2 in, 2 out]
          }
          frame "SwitchToMeas" {
            n112 = Get Date/Time In Seconds() -> (seconds since 1Jan1904=w329:timestamp)
            n113 = in-place {
              n114 = in-place-cluster #5(w331) -> ()  [unwired: 1 out]
              n115 = in-place-cluster #5("Operation.Operation Mode"=Mode_Enum."Idle") -> (w330:T7)
            }
            n116 = call "PromptWrite.vi"("error in"=w326, "time"=w329, "string"="Start Measuring... ", "TerminalIn"=w328) -> ("TerminalOut"=w325:T5)  [unwired: 6 in, 1 out]
            n117 = call "PassFailWrite.vi"("FailString"="Failed", "End"="\r\n", "PassString"="Success", "TerminalIn"=w325) -> ("error out"=w320:errorcluster, "TerminalOut"=w321:T5)  [unwired: 6 in]
            n118 = property on="Measuring" class="Bool (strict)"("Value"=TRUE ("Measuring")) -> ()  [unwired: 2 in, 2 out]
            n119 = property on="Logging" class="Bool (strict)"("Value"=FALSE ("Logging")) -> ()  [unwired: 2 in, 2 out]
          }
          frame "SwitchToLog" {
            (unwired) "Logging to File... " ("string")
            n120 = Get Date/Time In Seconds() -> (seconds since 1Jan1904=w346:timestamp)
            n121 = call "PromptWrite.vi"("error in"=w345, "time"=w346, "TerminalIn"=w347) -> ("error out"=w344:errorcluster, "TerminalOut"=w338:T5)  [unwired: 7 in]
            n122 = property on="Logging" class="Bool (strict)"("Value"=TRUE ("Logging")) -> ()  [unwired: 2 in, 2 out]
            n123 = property on="Measuring" class="Bool (strict)"("Value"=TRUE ("Measuring")) -> ()  [unwired: 2 in, 2 out]
            n124 = call "File Dialog"("prompt"="Where do you want to log measurements?", "error in"=w344) -> ("selected path"=w343:path, "cancelled"=w341:bool, "error out"=w339:errorcluster)  [unwired: 10 in, 1 out]
            n125 = in-place {
              in-place-border: w343 -> [w371]
              n126 = in-place-cluster #6(w349) -> ()  [unwired: 4 out]
              n127 = in-place-cluster #6("Operation.Operation Mode"=Mode_Enum."Logging", "Operation.Log Folder"=w371, "Timing.LastOp?"=FALSE, "Timing.FirstOp?"=TRUE) -> (w348:T7)
            }
            n128 = case shown="True" w341 {
              tunnel: w342 -> [_ w367]
              tunnel: w339 -> [w354 w365]
              tunnel: w338 -> [w356 w362]
              tunnel: [w353 w361] -> w337
              tunnel: [w355 w360] -> w336
              frame False {
                n129 = call "PassFailWrite.vi"("FailString"="Failed", "error in"=w354, "End"="\r\n", "PassString"="Ready", "TerminalIn"=w356) -> ("error out"=w353:errorcluster, "TerminalOut"=w355:T5)  [unwired: 5 in]
              }
              frame True {
                n130 = call "PassFailWrite.vi"("FailString"="Failed", "error in"=w365, "End"="\r\n", "PassString"="Cancelled", "TerminalIn"=w362) -> ("error out"=w361:errorcluster, "TerminalOut"=w360:T5)  [unwired: 5 in]
                n131 = Enqueue Element At Opposite End(queue=w367, element=cluster{T10, bool} {enum."SwitchToOff", FALSE}) -> ()  [unwired: 2 in, 3 out]
              }
            }
          }
          frame "UpdatePlots" {
            n132 = call "PlotHelper.vi"("Y-Axis"="Y-Axis", "X-Axis"="X-Axis", "Data_IN"=w383) -> ("Progress Plots"=→"Test Graph":cluster{"Variant X":dbl, "Variant Y":dbl}[], "Data_Out"=w378:T7)  [unwired: 7 in]
            n133 = property on="Test Graph" class="XYGraph (strict)"() -> ("Cursor.Cursor Index"=w377:i32)  [unwired: 2 in, 2 out]
            n134 = call "SelectSpectrum.vi"("Following"="Following", "Param"="Param", "Cursor.Cursor Index"=w377, "Data_IN"=w378) -> ("VNA Out"=→"Parameter Plots":cluster{"Ramp Pattern":dbl[], "VNA S22":dbl[]}, "Data_Out"=w374:T7)  [unwired: 6 in]
          }
          frame "RefreshPlotMUnits" {
            n135 = control-ref of="Parameter Plots"() -> (w386:refnum<vi>)
            n136 = control-ref of="Test Graph"() -> (w393:refnum<vi>)
            n137 = property on="Y-Axis" class="Enum (strict)"() -> ("Value"=w392:T3)  [unwired: 2 in, 2 out]
            n138 = property on="X-Axis" class="Enum (strict)"() -> ("Value"=w391:T3)  [unwired: 2 in, 2 out]
            n139 = property on="Param" class="Enum (strict)"() -> ("Value"=w387:enum16{"S11", "S21", "S12", "S22"})  [unwired: 2 in, 2 out]
            n140 = call "LCR_PlotNamer.vi"("Y-Axis"=w392, "X-Axis"=w391, "Param"=w387, "Parameter Plots"=w386, "T/B Ref In"=w393) -> ()  [unwired: 7 in]
          }
          frame "ClearBuffers" {
            n141 = in-place {
              n142 = in-place-cluster #7(w399) -> ("Measurements"=w401:T8[])
              n143 = Array Size(array=w401) -> (size(s)=w400:i32)
              n144 = Delete From Array(array=w401, length=w400, index=0) -> (array with subset deleted=w403:T8[])  [unwired: 1 out]
              n145 = in-place-cluster #7("Measurements"=w403) -> (w398:T7)
            }
          }
          frame "Disconnect" {
            n146 = Enqueue Element At Opposite End(queue=w409, element=cluster{T10, bool} {enum."ExitSafe", FALSE}, error in (no error)=w406) -> (error out=w404:errorcluster)  [unwired: 1 in, 2 out]
          }
          frame "ExitSafe" {
          }
        }
        n147 = call "GEN_CulArray.vi"("Max Values"="Max Elements", "Data_Cluster"=w113) -> ("Data_Cluster Out"=w112:T7)  [unwired: 9 in]
        n148 = Or(x=w110, y=w105) -> (x .or. y?=w116:bool)
      }
    }
    frame Error {
      n149 = control-ref of="Terminal"() -> ()  [unwired: 1 out]
      n150 = Unbundle By Name(w415) -> ()  [unwired: 1 out]
      n151 = flat-sequence {
        tunnel: w415 -> [w417]
        frame #0 {
          n152 = call <vilib>:"Clear Errors.vi"("error in (no error)"=w417) -> ()  [unwired: 5 in, 2 out]
        }
        frame #1 {
          n153 = Stop(stop? (T)=TRUE) -> ()
        }
      }
    }
  }
  n154 = property on="Measuring" class="Bool (strict)"("Colors [4]"=w31) -> ()  [unwired: 2 in, 2 out]
  n155 = property on="Logging" class="Bool (strict)"("Colors [4]"=w31) -> ()  [unwired: 2 in, 2 out]
  n156 = Generate User Event(user event=w21, event data cluster=TRUE, error in=w23) -> (user event out=w25:refnum<user-event>, error out=w24:errorcluster)  [unwired: 1 in]
  n157 = Destroy User Event(user event=w25, error in=w24) -> ()  [unwired: 1 out]
  "Global B" <- FALSE ("Globals")
  "Global T" <- FALSE ("HM 8118")
  "Logging" <- FALSE ("Logging")
  "Measuring" <- FALSE ("Measuring")
  "Terminal" <- w19
